vi "LIDAR_global.vi"() -> ()   [LabVIEW 2017]
panel:
  in  "LIDAR Angle (rad)":dbl[](array[numeric])
  in  "LIDAR Magnitude (m)":dbl[](array[numeric])
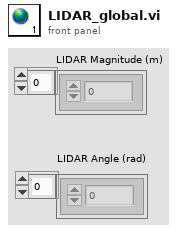
[diagram p1: front panel]
diagram:
